vi "Move Turret.vi"(7 "Mono System # (0)":T2, 8 "error in (no error)":errorcluster, 10 "turret position (default)":T1, 11 "VISA resource name":refnum<visa-resource-name>) -> (0 "error out":errorcluster, 3 "VISA resource name out":refnum<visa-resource-name>)   [LabVIEW 2009, in "JY-SPEX-TRIAX.lvlib"]
doc: "Moves the turret between the default setting (the one in use after initializing the spectrometer) and the \"other\" position."
uses:
  JY-SPEX-TRIAX.lvlib
  controls.llb/Monochromator System Number.ctl
  controls.llb/Turret Position.ctl
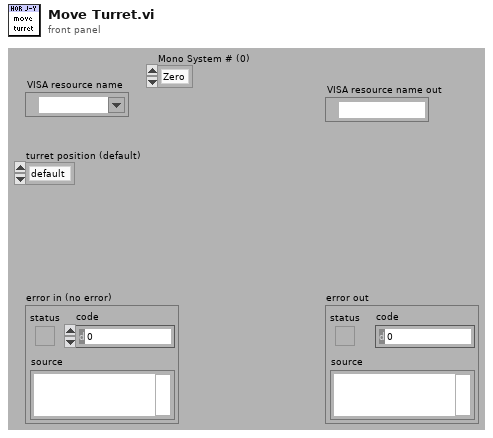
[diagram p1: front panel]
types:
  T1 = typedef "JY-SPEX-TRIAX.lvlib/Turret Position.ctl" = enum16{"default", "other"}
  T2 = typedef "JY-SPEX-TRIAX.lvlib/Monochromator System Number.ctl" = enum16{"Zero", "One"}
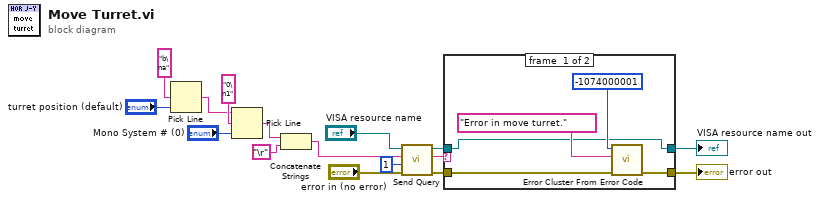
[diagram p0: block diagram]
diagram:
  n1 = Pick Line(multi-line string="b\na", line index="turret position (default)") -> (output string=w6:string)  [unwired: 1 out]
  n2 = Pick Line(string ("")=w6, multi-line string="0\n1", line index="Mono System # (0)") -> (output string=w4:string)
  n3 = Concatenate Strings(w4, "\r") -> (w2:string)
  n4 = call "Send Query.vi"("error in (no error)"="error in (no error)", "byte count"=u32 1, "write buffer"=w2, "VISA resource name"="VISA resource name") -> ("error out"=w9:errorcluster, "read buffer"=w12:string, "VISA resource name out"=w11:refnum<visa-resource-name>)  [unwired: 5 out]
  n5 = case shown="Default" w12 {
    tunnel: w11 -> [w17 w23]
    tunnel: [w17 w23] -> w10
    tunnel: w9 -> [w19 w22]
    tunnel: [w18 w22] -> w8
    frame #0 {
      n6 = call <vilib>:"Error Cluster From Error Code.vi"("error in (no error)"=w19, "error message (\"\")"="Error in move turret." ("error message (\"\")"), "error code (0)"=-1074000001) -> ("error out"=w18:errorcluster)  [unwired: 1 in, 5 out]
    }
    frame #1 {
    }
  }
  "VISA resource name out" <- w10
  "error out" <- w8
